vi "Genera e leggi due segnali due canali.vi"() -> ()   [LabVIEW 2014]
uses:
  <vilib>/measure/NI_MABase.lvlib
panel:
  out "Waveform Graph":dynamicdata(graph)
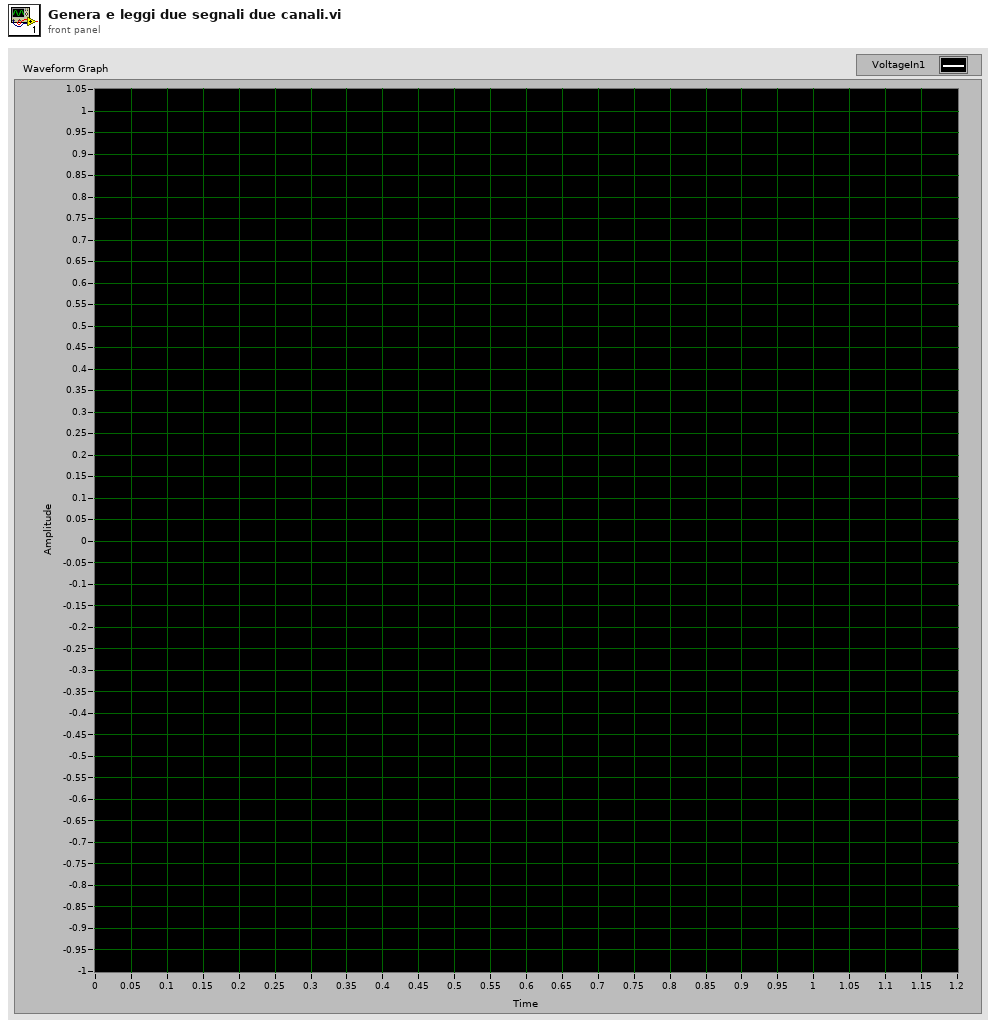
[diagram p1: front panel]
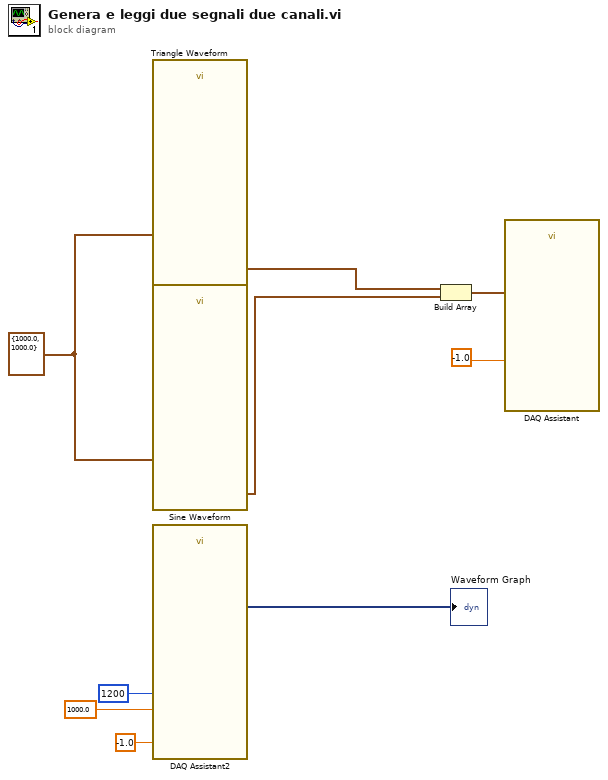
[diagram p0: block diagram]
diagram:
  w1 = cluster{"Fs":dbl, "#s":dbl} {"Fs"=1000.0, "#s"=1000.0} ("sampling info")
  n1 = call <vilib>:"Triangle Waveform.vi"("sampling info"=w1) -> ("signal out"=w5:waveform(dbl))  [unwired: 9 in, 1 out]
  n2 = call <vilib>:"Sine Waveform.vi"("sampling info"=w1) -> ("signal out"=w4:waveform(dbl))  [unwired: 9 in, 1 out]
  n3 = call "DAQ Assistant2"("rate"=1000.0, "number of samples"=1200, "timeout (s)"=-1.0) -> ("data"=→"Waveform Graph":dynamicdata)  [unwired: 14 in, 2 out]
  n4 = Build Array(w5, w4) -> (w3:waveform(dbl)[])
  n5 = call "DAQ Assistant"("data"=w3, "timeout (s)"=-1.0) -> ()  [unwired: 16 in, 2 out]
